vi "switchboard_query.vi"(8 "error in":errorcluster, 10 "Buffer":string="MATRIX.TEMPERATURE", 11 "Handle":u32) -> (0 "error out":errorcluster, 2 "Read Buffer Out":string, 3 "Handle":u32)   [LabVIEW 2016]
panel:
  out "This query return":string
  out "Full buffer content":string
  out "Bytes Read":u32
  out "Bytes Waiting":u32
  out "Bytes Written":u32
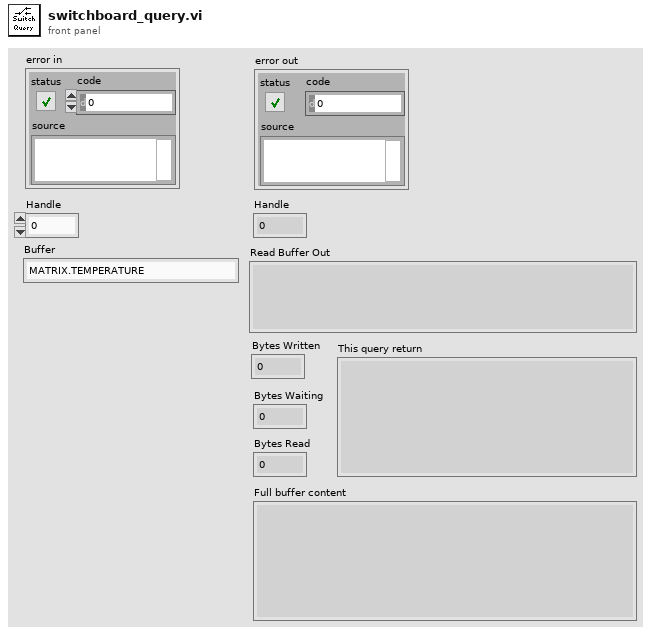
[diagram p1: front panel]
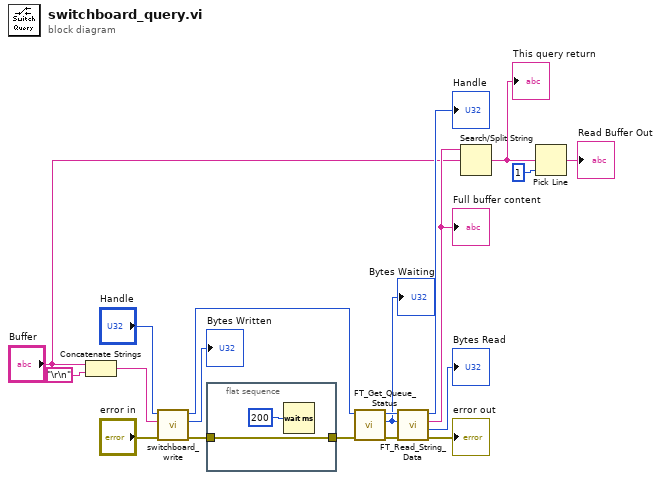
[diagram p0: block diagram]
diagram:
  n1 = Concatenate Strings("Buffer", "\r\n") -> (w8:string)
  n2 = call <instrlib>:"switchboard_write.vi"("error in"="error in", "Buffer"=w8, "Handle"="Handle") -> ("error out"=w6:errorcluster, "Bytes Written"=→"Bytes Written":u32, "Handle"=w4:u32)  [unwired: 6 in]
  n3 = flat-sequence {
    tunnel: w6 -> [w20]
    tunnel: [w20] -> w10
    frame #0 {
      n4 = Wait (ms)(milliseconds to wait=u32 200) -> ()  [unwired: 1 out]
    }
  }
  n5 = call <instrlib>:"FT_Get_Queue_Status.vi"("error in"=w10, "Handle"=w4) -> ("error out"=w16:errorcluster, "Bytes Waiting"=w18:u32, "Handle out"=w19:u32)  [unwired: 7 in]
  "Bytes Waiting" <- w18
  n6 = call <instrlib>:"FT_Read_String_Data.vi"("error in"=w16, "Bytes To Read"=w18, "Handle"=w19) -> ("error out"=→"error out":errorcluster, "Bytes Read"=→"Bytes Read":u32, "Read Data"=w3:string, "Handle out"=→"Handle":u32)  [unwired: 5 in]
  "Full buffer content" <- w3
  n7 = Search/Split String(string=w3, search string/char (-)="Buffer") -> (match + rest of string=w1:string)  [unwired: 1 in, 2 out]
  "This query return" <- w1
  n8 = Pick Line(multi-line string=w1, line index=1) -> (output string=→"Read Buffer Out":string)  [unwired: 1 in]
